vi "Drive Train.vi"() -> ()   [LabVIEW 2018]
uses:
  <vilib>/Rock Robotics/SystemInterfaces/DIO/FPGA_DIOChannel.ctl
  <vilib>/Rock Robotics/SystemInterfaces/AI/FPGA_AIChannel.ctl
  <vilib>/Rock Robotics/WPI/ThirdParty/Sensors/navX/_TypeDefs/FRIC_navX_DeviceNumbersTypeDef.ctl
  <vilib>/Rock Robotics/WPI/ThirdParty/Phoenix-LabVIEW/Motor Controller/Controls/CTRE_Phoenix_MotorControl_NeutralMode.ctl
  <vilib>/Rock Robotics/WPI/Counter/WPI_CounterDigitalInputToDigitalSource.vi
  Times/Times Global.vi
  Drive Train Global.vi
  <vilib>/ptbypt/NI_PtbyPt.lvlib
panel:
  out "Cont Yaw Zero":dbl
  out "Loop 2":u32=30
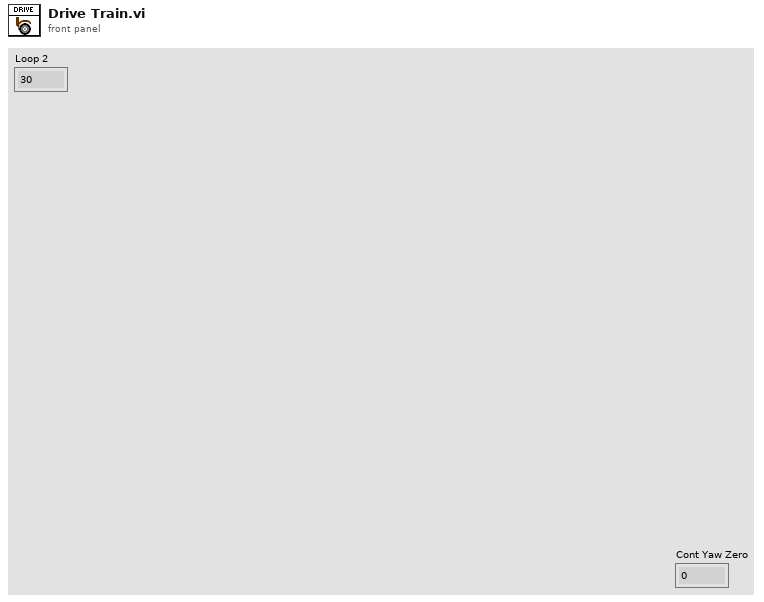
[diagram p1: front panel]
types:
  T1 = typedef "FPGA_AIChannel.ctl" = enum8{"AI 0", "AI 1", "AI 2", "AI 3", "AI MXP 0", "AI MXP 1", "AI MXP 2", "AI MXP 3", "Invalid"}
  T2 = typedef "FPGA_DIOChannel.ctl" = enum8{"DIO 0", "DIO 1", "DIO 2", "DIO 3", "DIO 4", "DIO 5", "DIO 6", "DIO 7", "DIO 8", "DIO 9", "DIO MXP 0", "DIO MXP 1", "DIO MXP 2", "DIO MXP 3", "DIO MXP 4", "DIO MXP 5", "DIO MXP 6", "DIO MXP 7", "DIO MXP 8", "DIO MXP 9", "DIO MXP 10", "DIO MXP 11", "DIO MXP 12", "DIO MXP 13", "DIO MXP 14", "DIO MXP 15", "SPI Port CS1", "SPI Port CS2", "SPI Port CS3", "SPI Port MISO", "SPI Port MOSI", "Invalid"}
  T3 = typedef "FRIC_navX_DeviceNumbersTypeDef.ctl" = enum16{"Dev0", "Dev1", "Dev2", "Dev3"}
  T4 = cluster{"Rollover":dbl, "Yaw":dbl, "Cont Yaw":dbl}
  T5 = typedef "Control 2.ctl" = dbl
  T6 = typedef "CTRE_Phoenix_MotorControl_NeutralMode.ctl" = enum8{"EEPROMSetting", "Override to Coast", "Override to Brake"}
  T7 = typedef "WPI_MotorControlDeviceRef.ctl" = cluster{"DeviceStatus":errorcluster, "Type":T8, "PWM":cluster{"PWM Channel":T9, "DeadBand":T10}, "CAN":cluster{"Device Number":u8, "SetOutput VI Ref":variant, "GetOutput VI Ref":variant, "Enable VI Ref":variant, "Disable VI Ref":variant, "Data":variant}, "Invert":bool, "DIO PWM":cluster{"PWM \"Enable\" Channel":T9, "DIOChannel":T2, "PWM Rate":dbl}}
  T8 = typedef "WPI_MotorControlType.ctl" = enum16{"PWM", "CAN", "DIO PWM"}
  T9 = typedef "FPGA_DIOPWMChannel.ctl" = enum8{"PWM 0", "PWM 1", "PWM 2", "PWM 3", "PWM 4", "PWM 5", "PWM 6", "PWM 7", "PWM 8", "PWM 9", "PWM MXP 0", "PWM MXP 1", "PWM MXP 2", "PWM MXP 3", "PWM MXP 4", "PWM MXP 5", "PWM MXP 6", "PWM MXP 7", "PWM MXP 8", "PWM MXP 9", "Invalid"}
  T10 = typedef "WPI_PWMDeadband.ctl" = cluster{"Name":string, "maxPositivePwm":i32, "minPositivePwm":i32, "centerPwm":i32, "maxNegativePwm":i32, "minNegativePwm":i32, "angularRange":u16}
  T11 = typedef "WPI_DigitalInputDevRef.ctl" = cluster{"DevStatus":errorcluster, "DIO Channel":T2}
  T12 = typedef "WPI_PotentiometerDevRef.ctl" = cluster{"DevStatus":errorcluster, "Analog Channel":T1, "Invert Output":bool}
  T13 = typedef "FPGA_CounterEncoderSourceConvertionLVSourceType.ctl" = cluster{"DevStatus":errorcluster, "AnalogTriggerMode?":bool, "DigitalMode":cluster{"DIO Channel":T14}, "AnalogTriggerMode":cluster{"AnalogTriggerIndex":T15, "OutputType":T16}}
  T14 = typedef "FPGA_DIODigitalSourceChannel.ctl" = enum8{"DIO 0", "DIO 1", "DIO 2", "DIO 3", "DIO 4", "DIO 5", "DIO 6", "DIO 7", "DIO 8", "DIO 9", "DIO MXP 0", "DIO MXP 1", "DIO MXP 2", "DIO MXP 3", "DIO MXP 4", "DIO MXP 5", "DIO MXP 6", "DIO MXP 7", "DIO MXP 8", "DIO MXP 9", "DIO MXP 10", "DIO MXP 11", "DIO MXP 12", "DIO MXP 13", "DIO MXP 14", "DIO MXP 15", "SPI Port CS1", "SPI Port CS2", "SPI Port CS3", "SPI Port MISO", "SPI Port MOSI", "Disabled"}
  T15 = typedef "FPGA_AnalogTriggerIndex.ctl" = enum8{"Trig 0", "Trig 1", "Trig 2", "Trig 3", "Trig 4", "Trig 5", "Trig 6", "Trig 7", "Invalid"}
  T16 = typedef "FPGA_AnalogTriggerOutType.ctl" = enum16{"InWindow", "TriggerState", "Rising", "Falling"}
  T17 = typedef "WPI_EncoderDevRef.ctl" = cluster{"DevStatus":errorcluster, "EncoderIndex":T18, "CounterIndex":T19, "DistancePerCount":dbl, "Decoding Type":T20}
  T18 = typedef "FPGA_EncoderIdx.ctl" = enum8{"Enc 0", "Enc 1", "Enc 2", "Enc 3", "Enc 4", "Enc 5", "Enc 6", "Enc 7", "Invalid"}
  T19 = typedef "FPGA_CounterCtrSystemIndex.ctl" = enum8{"Ctr 0", "Ctr 1", "Ctr 2", "Ctr 3", "Ctr 4", "Ctr 5", "Ctr 6", "Ctr 7", "Invalid"}
  T20 = typedef "WPI_EncoderType.ctl" = enum16{"1x", "2x", "4x"}
  T21 = cluster{"FrontLeft":dbl, "FrontRight":dbl, "BackLeft":dbl, "BackRight":dbl}
  T22 = enum16{"Back Left", "Back Right", "Front Left", "Front Right"}
  T23 = enum16{"Autonomous Mode", "Field Oriented", "Robot Oriented", "Tank Mode"}
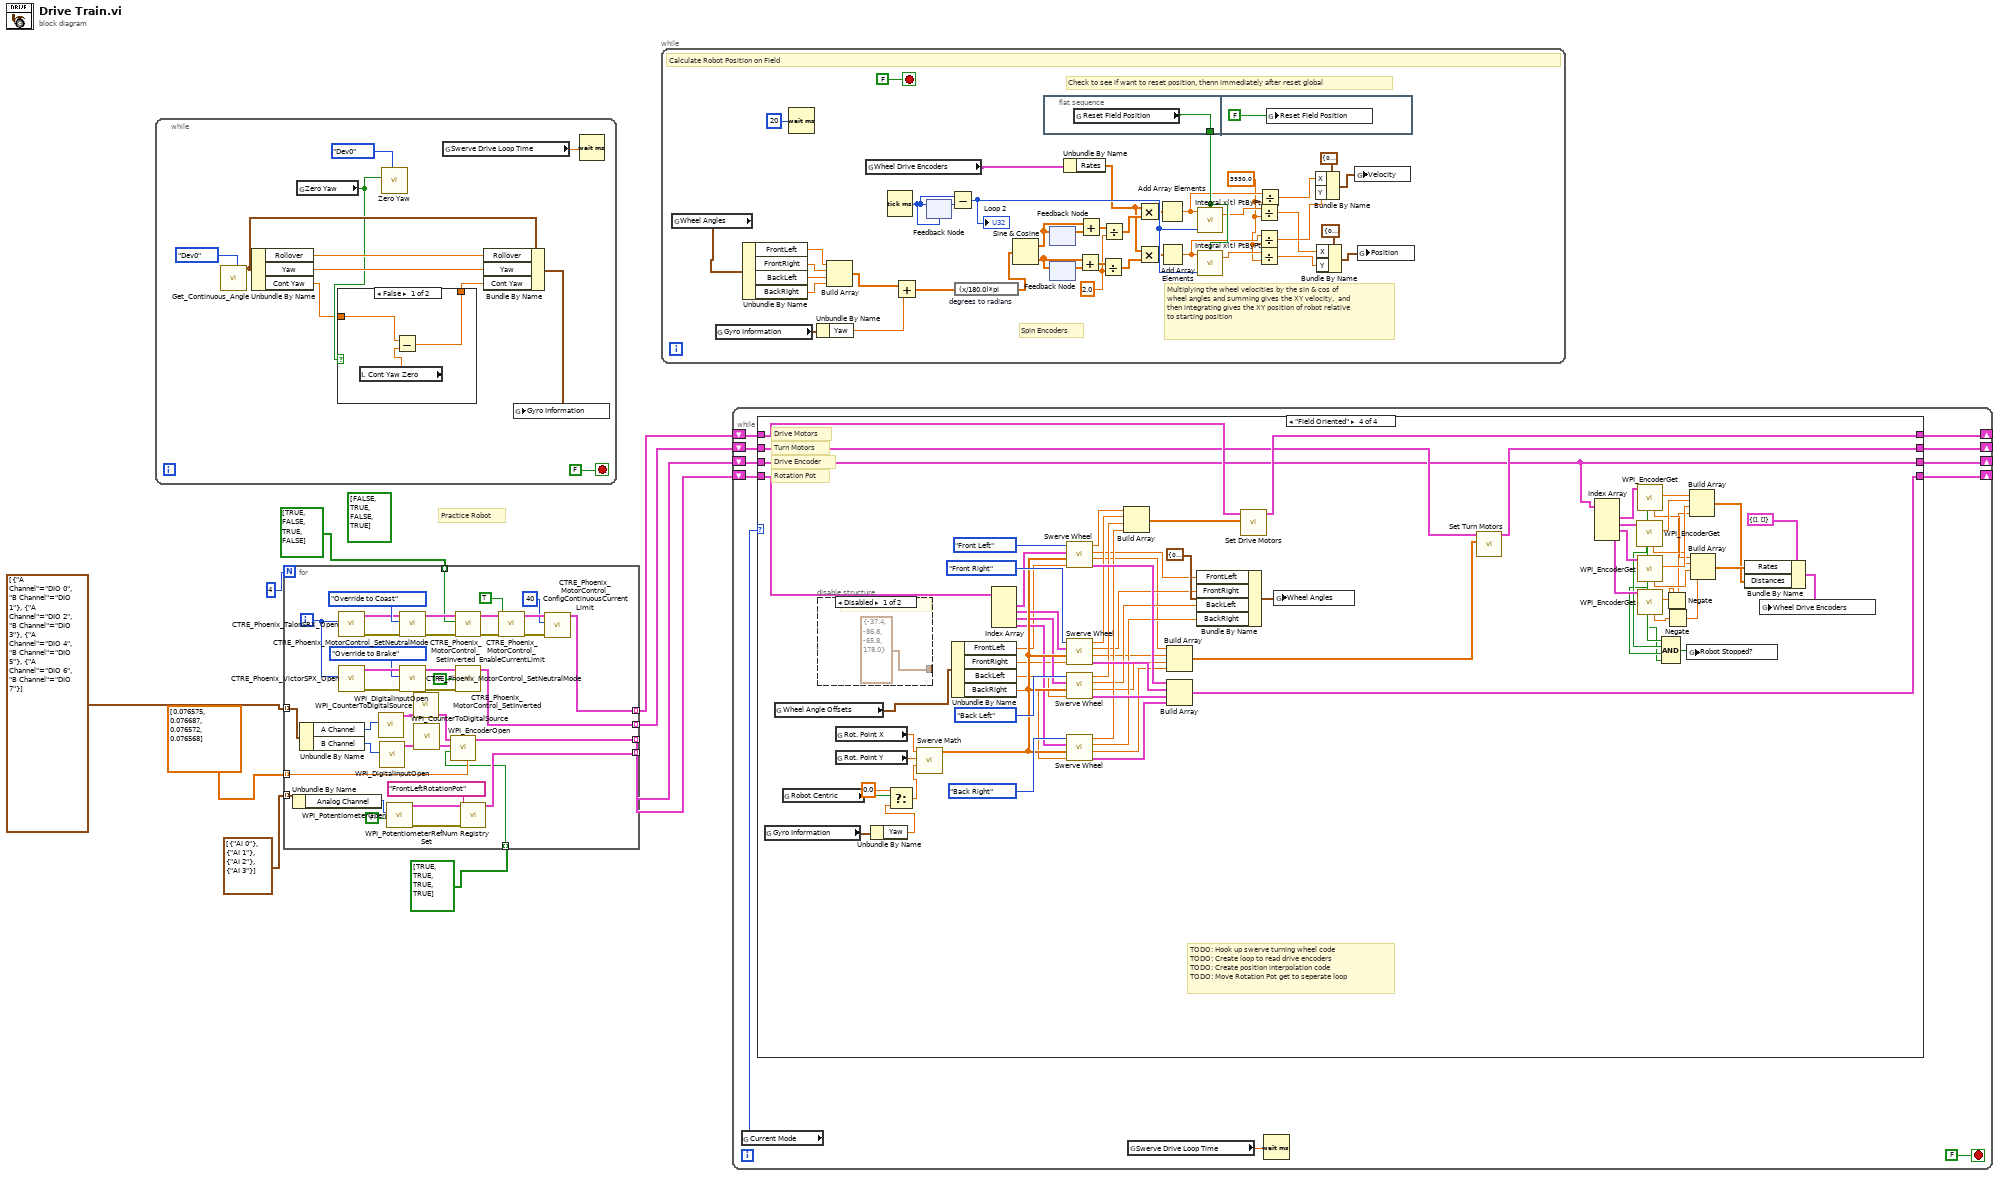
[diagram p0: block diagram]
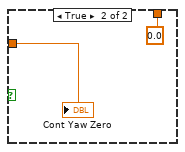
[diagram p2: hidden frame]
diagram:
  (unwired) bool[] [FALSE, TRUE, FALSE, TRUE]
  # "Practice Robot"
  n1 = while {
    stop <- FALSE stop-if-true
    n2 = call <vilib>:"Get_Continuous_Angle.vi"("Device Number"=FRIC_navX_DeviceNumbersTypeDef."Dev0") -> ("Continuous Angle"=w15:T4)  [unwired: 10 in]
    n3 = Unbundle By Name(w15) -> ("Rollover"=w16:dbl, "Yaw"=w14:dbl, "Cont Yaw"=w12:dbl)
    n4 = global read "Drive Train Global.vi" "Zero Yaw"() -> (w13:bool)
    n5 = case shown="False" w13 {
      tunnel: w12 -> [w24 w26]
      tunnel: [w23 0.0] -> w11
      frame False {
        n6 = local read "Cont Yaw Zero"() -> (w22:dbl)
        n7 = Subtract(x=w24, y=w22) -> (x-y=w23:dbl)
      }
      frame True {
        "Cont Yaw Zero" <- w26
      }
    }
    n8 = call <vilib>:"Zero Yaw.vi"("Device Number"=FRIC_navX_DeviceNumbersTypeDef."Dev0", "Zero"=w13) -> ()  [unwired: 10 in]
    n9 = global read "Times Global.vi" "Swerve Drive Loop Time"() -> (w19:T5)
    n10 = Bundle By Name(cluster=w15, "Rollover"=w16, "Yaw"=w14, "Cont Yaw"=w11) -> (w17:T4)
    n11 = global write "Drive Train Global.vi" "Gyro Information"(w17) -> ()
    n12 = Wait (ms)(milliseconds to wait=w19) -> ()  [unwired: 1 out]
  }
  n13 = for {
    N: 4 -> [_]
    tunnel: cluster{"A Channel":T2, "B Channel":T2}[] [{"A Channel"=enum."DIO 0", "B Channel"=enum."DIO 1"}, {"A Channel"=enum."DIO 2", "B Channel"=enum."DIO 3"}, {"A Channel"=enum."DIO 4", "B Channel"=enum."DIO 5"}, {"A Channel"=enum."DIO 6", "B Channel"=enum."DIO 7"}] -> [w44] mode=indexing
    tunnel: cluster{"Analog Channel":T1}[] [{"Analog Channel"=enum."AI 0"}, {"Analog Channel"=enum."AI 1"}, {"Analog Channel"=enum."AI 2"}, {"Analog Channel"=enum."AI 3"}] -> [w41] mode=indexing
    tunnel: dbl[] [0.076575, 0.076687, 0.076572, 0.076568] -> [w39] mode=indexing
    tunnel: [w28] -> w6 mode=indexing
    tunnel: [w38] -> w5 mode=indexing
    tunnel: [w37] -> w4 mode=indexing
    tunnel: [w36] -> w3 mode=indexing
    tunnel: bool[] [TRUE, FALSE, TRUE, FALSE] -> [w35] mode=indexing
    tunnel: bool[] [TRUE, TRUE, TRUE, TRUE] -> [w27] mode=indexing
    i -> [w45]
    n14 = Unbundle By Name(w41) -> ("Analog Channel"=w40:T1)
    n15 = Unbundle By Name(w44) -> ("A Channel"=w43:T2, "B Channel"=w42:T2)
    n16 = call <vilib>:"CTRE_Phoenix_TalonSRX_Open.vi"("Device Number"=w45) -> ("error out"=w46:errorcluster, "CAN Talon SRX Ref"=w47:T7)  [unwired: 9 in]
    n17 = call <vilib>:"CTRE_Phoenix_VictorSPX_Open.vi"("Device Number"=w45) -> ("error out"=w56:errorcluster, "CAN Talon SRX Ref"=w55:T7)  [unwired: 9 in]
    n18 = call <vilib>:"WPI_DigitalInputOpen.vi"("DIO Channel"=w43) -> ("DigitalInputDevRef"=w63:T11)  [unwired: 1 in, 9 out]
    n19 = call <vilib>:"WPI_DigitalInputOpen.vi"("DIO Channel"=w42) -> ("DigitalInputDevRef"=w62:T11)  [unwired: 1 in, 9 out]
    n20 = call <vilib>:"WPI_PotentiometerOpen.vi"("Invert Output"=FALSE, "Analog Channel"=w40) -> ("error out"=w58:errorcluster, "PotDevRef"=w59:T12)  [unwired: 8 in]
    n21 = call <vilib>:"CTRE_Phoenix_MotorControl_SetNeutralMode.vi"("error in (no error)"=w46, "Motor Control Neutral Mode"=CTRE_Phoenix_MotorControl_NeutralMode."Override to Coast", "PhoenixMotorControlDevRef"=w47) -> ("error out"=w49:errorcluster, "PhoenixMotorControlDevRef"=w50:T7)  [unwired: 7 in]
    n22 = call <vilib>:"CTRE_Phoenix_MotorControl_SetNeutralMode.vi"("error in (no error)"=w56, "Motor Control Neutral Mode"=CTRE_Phoenix_MotorControl_NeutralMode."Override to Brake", "PhoenixMotorControlDevRef"=w55) -> ("error out"=w53:errorcluster, "PhoenixMotorControlDevRef"=w52:T7)  [unwired: 7 in]
    n23 = call-poly <vilib>:"WPI_CounterToDigitalSource.vi"("DigitalInputDevRef"=w63) -> ("Digital Source"=w64:T13)  [unwired: 6 out]
    n24 = call-poly <vilib>:"WPI_CounterToDigitalSource.vi"("DigitalInputDevRef"=w62) -> ("Digital Source"=w61:T13)  [unwired: 6 out]
    n25 = call <vilib>:"WPI_EncoderOpen.vi"("DistancePerCount"=w39, "Invert Direction (False)"=w27, "BSource"=w61, "ASource"=w64) -> ("EncoderDevRef"=w37:T17)  [unwired: 4 in, 3 out]
    n26 = call <vilib>:"CTRE_Phoenix_MotorControl_SetInverted.vi"("error in (no error)"=w49, "Invert?"=w35, "PhoenixMotorControlDevRef"=w50) -> ("error out"=w34:errorcluster, "PhoenixMotorControlDevRef"=w33:T7)  [unwired: 7 in]
    n27 = call <vilib>:"CTRE_Phoenix_MotorControl_SetInverted.vi"("error in (no error)"=w53, "Invert?"=FALSE, "PhoenixMotorControlDevRef"=w52) -> ("PhoenixMotorControlDevRef"=w38:T7)  [unwired: 7 in, 1 out]
    n28 = call <vilib>:"WPI_PotentiometerRefNum Registry Set.vi"("error in (no error)"=w58, "refnum name"="FrontLeftRotationPot", "PotDevRef"=w59) -> ("PotDevRef"=w36:T12)  [unwired: 7 in, 1 out]
    n29 = call <vilib>:"CTRE_Phoenix_MotorControl_EnableCurrentLimit.vi"("error in (no error)"=w34, "Enable Current Limit?"=TRUE, "PhoenixMotorControlDevRef"=w33) -> ("error out"=w31:errorcluster, "PhoenixMotorControlDevRef"=w30:T7)  [unwired: 7 in]
    n30 = call <vilib>:"CTRE_Phoenix_MotorControl_ConfigContinuousCurrentLimit.vi"("error in (no error)"=w31, "Continuous Current Limit (Amps)"=40, "PhoenixMotorControlDevRef"=w30) -> ("PhoenixMotorControlDevRef"=w28:T7)  [unwired: 7 in, 1 out]
  }
  n31 = while {
    stop <- FALSE stop-if-true
    w84 = 3930.0 ("y")
    w95 = 2.0
    # "Check to see if want to reset position, thenn immediately after reset global"
    # "Spin Encoders"
    # "Multiplying the wheel velocities by the sin & cos of wheel angles and summing gives the XY velocity,  and then integrating gives the XY position of robot relative to starting position"
    # "Calculate Robot Position on Field"
    n32 = global read "Drive Train Global.vi" "Wheel Angles"() -> (w82:T21)
    n33 = global read "Drive Train Global.vi" "Gyro Information"() -> (w75:T4)
    n34 = Unbundle By Name(w82) -> ("FrontLeft"=w81:dbl, "FrontRight"=w80:dbl, "BackLeft"=w79:dbl, "BackRight"=w78:dbl)
    n35 = Wait (ms)(milliseconds to wait=u32 20) -> ()  [unwired: 1 out]
    n36 = Unbundle By Name(w75) -> ("Yaw"=w74:dbl)
    n37 = Build Array(w81, w80, w79, w78) -> (w77:dbl[])
    n38 = global read "Drive Train Global.vi" "Wheel Drive Encoders"() -> (w76:cluster{"Rates":dbl[], "Distances":dbl[]})
    n39 = Tick Count (ms)() -> (millisecond timer value=w90:u32)
    n40 = Add(x=w77, y=w74) -> (x+y=w83:dbl[])
    n41 = feedback #1(w90) -> (w106:u32)
    n42 = feedback-in #1(w90) -> ()
    n43 = Subtract(x=w90, y=w106) -> (x-y=w105:u32)
    "Loop 2" <- w105
    n44 = expression code="(x/180.0)*pi" "degrees to radians"(w83) -> (w89:dbl[])
    n45 = Sine & Cosine(0:w89) -> (1:w101:dbl[], 2:w96:dbl[])
    n46 = flat-sequence {
      tunnel: [w107] -> w92
      frame #0 {
        n47 = global read "Drive Train Global.vi" "Reset Field Position"() -> (w107:bool)
      }
      frame #1 {
        n48 = global write "Drive Train Global.vi" "Reset Field Position"(FALSE) -> ()
      }
    }
    n49 = feedback #2() -> (w102:dbl[])  [unwired: 1 in]
    n50 = feedback-in #2(w101) -> ()
    n51 = feedback #3() -> (w97:dbl[])  [unwired: 1 in]
    n52 = feedback-in #3(w96) -> ()
    n53 = Unbundle By Name(w76) -> ("Rates"=w91:dbl[])
    n54 = Add(x=w96, y=w97) -> (x+y=w98:dbl[])
    n55 = Add(x=w101, y=w102) -> (x+y=w99:dbl[])
    n56 = Divide(x=w98, y=w95) -> (x/y=w94:dbl[])
    n57 = Divide(x=w99, y=w95) -> (x/y=w100:dbl[])
    n58 = Multiply(x=w91, y=w100) -> (x*y=w104:dbl[])
    n59 = Multiply(x=w91, y=w94) -> (x*y=w103:dbl[])
    n60 = Add Array Elements(numeric array=w104) -> (sum=w87:dbl)
    n61 = Add Array Elements(numeric array=w103) -> (sum=w86:dbl)
    n62 = call <vilib>:"Integral x(t) PtByPt.vi"("initialize"=w92, "dt"=w105, "x"=w87) -> ("integral x(t)"=w88:dbl)  [unwired: 1 in, 1 out]
    n63 = call <vilib>:"Integral x(t) PtByPt.vi"("initialize"=w92, "dt"=w105, "x"=w86) -> ("integral x(t)"=w85:dbl)  [unwired: 1 in, 1 out]
    n64 = Divide(x=w88, y=w84) -> (x/y=w68:dbl)
    n65 = Divide(x=w86, y=w84) -> (x/y=w71:dbl)
    n66 = Divide(x=w85, y=w84) -> (x/y=w67:dbl)
    n67 = Divide(x=w87, y=w84) -> (x/y=w73:dbl)
    n68 = Bundle By Name(cluster=cluster{"X":dbl, "Y":dbl} {"X"=0.0, "Y"=0.0} ("Position"), "X"=w73, "Y"=w71) -> (w65:cluster{"X":dbl, "Y":dbl})
    n69 = Bundle By Name(cluster=cluster{"X":dbl, "Y":dbl} {"X"=0.0, "Y"=0.0} ("Position"), "X"=w68, "Y"=w67) -> (w69:cluster{"X":dbl, "Y":dbl})
    n70 = global write "Drive Train Global.vi" "Velocity"(w65) -> ()
    n71 = global write "Drive Train Global.vi" "Position"(w69) -> ()
  }
  n72 = while {
    shift-right: [w112] -> _
    shift-left: w6 -> [w116]
    shift-right: [w111] -> _
    shift-left: w5 -> [w115]
    shift-right: [w110] -> _
    shift-left: w4 -> [w114]
    shift-right: [w109] -> _
    shift-left: w3 -> [w113]
    stop <- FALSE stop-if-true
    n73 = global read "Drive Train Global.vi" "Current Mode"() -> (w117:T23)
    n74 = case shown="\"Field Oriented\"" w117 {
      tunnel: w116 -> [w123 w127 w131 w180]
      tunnel: w115 -> [w122 w126 w130 w168]
      tunnel: w114 -> [w121 w125 w129 w155]
      tunnel: w113 -> [w120 w124 w128 w190]
      tunnel: [w123 w127 w131 w179] -> w112
      tunnel: [w122 w126 w130 w167] -> w111
      tunnel: [w121 w125 w129 w155] -> w110
      tunnel: [w120 w124 w128 w189] -> w109
      frame "Autonomous Mode", Default {
        # "Rotation Pot"
        # "Drive Encoder"
        # "Turn Motors"
        # "Drive Motors"
      }
      frame "Robot Oriented" {
        # "Rotation Pot"
        # "Drive Encoder"
        # "Turn Motors"
        # "Drive Motors"
      }
      frame "Tank Mode" {
        # "Rotation Pot"
        # "Drive Encoder"
        # "Turn Motors"
        # "Drive Motors"
      }
      frame "Field Oriented" {
        # "TODO: Hook up swerve turning wheel code\nTODO: Create loop to read drive encoders\nTODO: Create position interpolation code\nTODO: Move Rotation Pot get to seperate loop"
        # "Rotation Pot"
        # "Drive Encoder"
        # "Turn Motors"
        # "Drive Motors"
        n75 = global read "Drive Train Global.vi" "Gyro Information"() -> (w197:T4)
        n76 = global read "Drive Train Global.vi" "Wheel Angle Offsets"() -> (w158:T21)
        n77 = global read "Drive Train Global.vi" "Robot Centric"() -> (w161:bool)
        n78 = disable-structure shown="Disabled" {
          disable-tunnel: [T21 {"FrontLeft"=-37.4, "FrontRight"=-86.8, "BackLeft"=-65.8, "BackRight"=178.0} ("Wheel Angle Offsets") _] -> _
          frame Disabled {
            # "Wheel Angle Offsets"
          }
          frame Enabled {
          }
        }
        n79 = global read "Drive Train Global.vi" "Rot. Point X"() -> (w196:dbl)
        n80 = global read "Drive Train Global.vi" "Rot. Point Y"() -> (w195:dbl)
        n81 = Unbundle By Name(w197) -> ("Yaw"=w159:dbl)
        n82 = Select(t=0.0, s=w161, f=w159) -> (s? t:f=w162:dbl)
        n83 = call "Swerve Math.vi"("Yaw"=w162, "Rot. Point Y"=w195, "Rot. Point X"=w196) -> ("Swerve Math Ouput"=w198:dbl[])  [unwired: 8 in]
        n84 = Unbundle By Name(w158) -> ("FrontLeft"=w166:dbl, "FrontRight"=w165:dbl, "BackLeft"=w164:dbl, "BackRight"=w163:dbl)
        n85 = Index Array(array=w190) -> (element #1=w194:T12, element #2=w193:T12, element #3=w192:T12, element #4=w191:T12)  [unwired: 4 in]
        n86 = call "Swerve Wheel.vi"("Wheel Angle Offset"=w166, "Inputs"=w198, "Pot Ref In"=w194, "Wheel"=T22."Front Left") -> ("Pot Ref Out"=w185:T12, "Motor Output"=w172:dbl, "Wheel Angle"=w177:dbl, "Speed"=w184:dbl)  [unwired: 4 in]
        n87 = call "Swerve Wheel.vi"("Wheel Angle Offset"=w165, "Inputs"=w198, "Pot Ref In"=w193, "Wheel"=T22."Front Right") -> ("Pot Ref Out"=w186:T12, "Motor Output"=w171:dbl, "Wheel Angle"=w176:dbl, "Speed"=w183:dbl)  [unwired: 4 in]
        n88 = call "Swerve Wheel.vi"("Wheel Angle Offset"=w164, "Inputs"=w198, "Pot Ref In"=w192, "Wheel"=T22."Back Left") -> ("Pot Ref Out"=w187:T12, "Motor Output"=w170:dbl, "Wheel Angle"=w175:dbl, "Speed"=w182:dbl)  [unwired: 4 in]
        n89 = call "Swerve Wheel.vi"("Wheel Angle Offset"=w163, "Inputs"=w198, "Pot Ref In"=w191, "Wheel"=T22."Back Right") -> ("Pot Ref Out"=w188:T12, "Motor Output"=w169:dbl, "Wheel Angle"=w174:dbl, "Speed"=w181:dbl)  [unwired: 4 in]
        n90 = Build Array(w184, w183, w182, w181) -> (w156:dbl[])
        n91 = Build Array(w172, w171, w170, w169) -> (w157:dbl[])
        n92 = Build Array(w185, w186, w187, w188) -> (w189:T12[])
        n93 = Bundle By Name(cluster=T21 {"FrontLeft"=0.0, "FrontRight"=0.0, "BackLeft"=0.0, "BackRight"=0.0} ("Wheel Angles"), "FrontLeft"=w177, "FrontRight"=w176, "BackLeft"=w175, "BackRight"=w174) -> (w173:T21)
        n94 = call "Set Drive Motors.vi"("appended array"=w156, "Motors In"=w180) -> ("Motors Out"=w179:T7[])  [unwired: 9 in]
        n95 = global write "Drive Train Global.vi" "Wheel Angles"(w173) -> ()
        n96 = call "Set Turn Motors.vi"("appended array"=w157, "Motors In"=w168) -> ("Motors Out"=w167:T7[])  [unwired: 9 in]
        n97 = Index Array(array=w155) -> (element #1=w154:T17, element #2=w153:T17, element #3=w152:T17, element #4=w151:T17)  [unwired: 4 in]
        n98 = call <vilib>:"WPI_EncoderGet.vi"("EncoderDevRef"=w153) -> ("Distance"=w147:dbl, "Rate"=w144:dbl, "Stopped"=w138:bool)  [unwired: 5 in, 3 out]
        n99 = call <vilib>:"WPI_EncoderGet.vi"("EncoderDevRef"=w154) -> ("Distance"=w148:dbl, "Rate"=w145:dbl, "Stopped"=w139:bool)  [unwired: 5 in, 3 out]
        n100 = call <vilib>:"WPI_EncoderGet.vi"("EncoderDevRef"=w152) -> ("Distance"=w146:dbl, "Rate"=w143:dbl, "Stopped"=w137:bool)  [unwired: 5 in, 3 out]
        n101 = call <vilib>:"WPI_EncoderGet.vi"("EncoderDevRef"=w151) -> ("Distance"=w133:dbl, "Rate"=w134:dbl, "Stopped"=w136:bool)  [unwired: 5 in, 3 out]
        n102 = Compound Arithmetic op=AND(w139, w138, w137, w136) -> (w140:bool)
        n103 = Negate(x=w133) -> (-x=w132:dbl)
        n104 = Negate(x=w134) -> (-x=w135:dbl)
        n105 = global write "Drive Train Global.vi" "Robot Stopped?"(w140) -> ()
        n106 = Build Array(w148, w147, w146, w132) -> (w141:dbl[])
        n107 = Build Array(w145, w144, w143, w135) -> (w142:dbl[])
        n108 = Bundle By Name(cluster=cluster{"Rates":dbl[], "Distances":dbl[]} {"Rates"=[], "Distances"=[]} ("Wheel Drive Encoders"), "Rates"=w142, "Distances"=w141) -> (w150:cluster{"Rates":dbl[], "Distances":dbl[]})
        n109 = global write "Drive Train Global.vi" "Wheel Drive Encoders"(w150) -> ()
      }
    }
    n110 = global read "Times Global.vi" "Swerve Drive Loop Time"() -> (w118:T5)
    n111 = Wait (ms)(milliseconds to wait=w118) -> ()  [unwired: 1 out]
  }
